vi "IGene_GetType.vi"(8 "error in":errorcluster, 11 "IGene in":refnum<class "IGene.lvclass">) -> (0 "error out":errorcluster, 3 "IGene out":refnum<class "IGene.lvclass">)   [LabVIEW 2016, in "IGene.lvclass"]
uses:
  IGene.lvclass
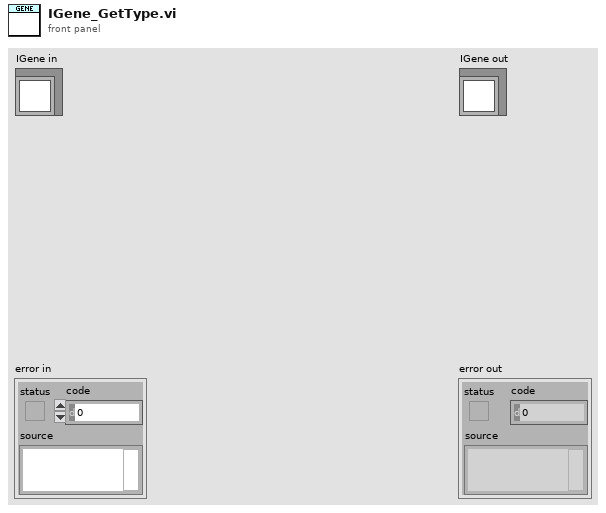
[diagram p1: front panel]
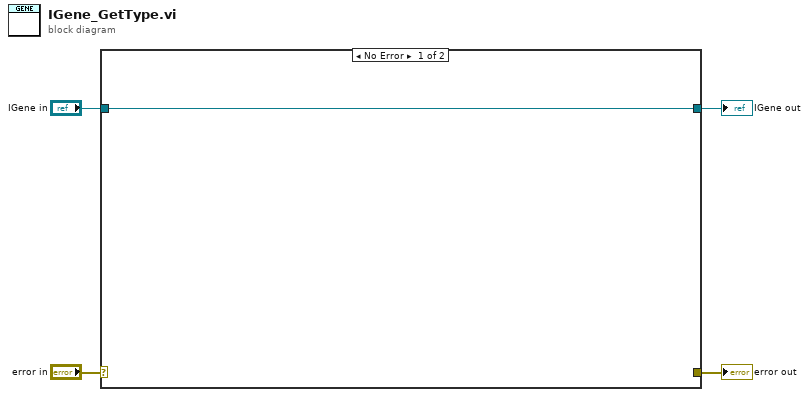
[diagram p0: block diagram]
diagram:
  n1 = case shown="No Error" "error in" {
    selector: "error in" -> [_ w7]
    tunnel: [_ w7] -> w3
    tunnel: [w5 w6] -> w1
    tunnel: "IGene in" -> [w5 w6]
    frame No Error {
    }
    frame Error {
    }
  }
  "error out" <- w3
  "IGene out" <- w1
